vi "Serial Write.vi"(8 "error in (no error)":errorcluster, 9 "Write Buffer":string, 10 "Connection ID":i32, 11 "Gantry in":refnum<class "Gantry.lvclass">) -> (0 "error out":errorcluster, 2 "Bytes written":u32, 3 "Gantry out":refnum<class "Gantry.lvclass">)   [LabVIEW 2023, in "Gantry.lvclass"]
uses:
  Gantry.lvclass
  Gantry.lvclass/Gantry.ctl
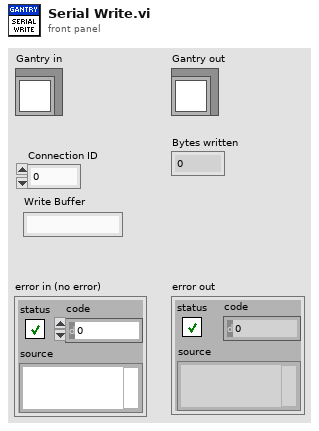
[diagram p1: front panel]
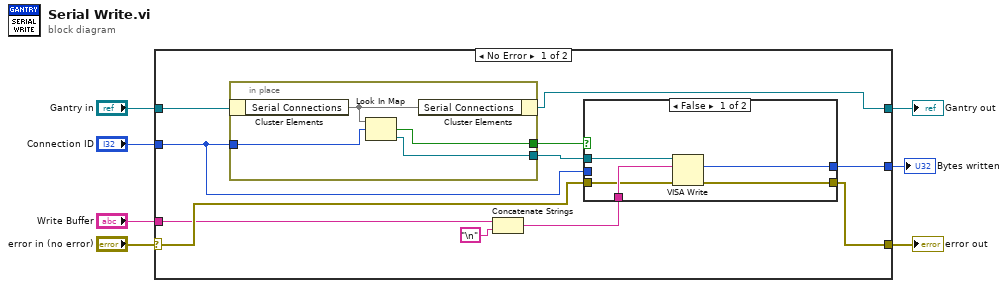
[diagram p0: block diagram]
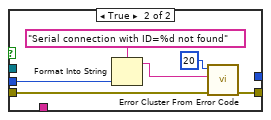
[diagram p2: hidden frame]
diagram:
  n1 = case shown="No Error" "error in (no error)" {
    selector: "error in (no error)" -> [w13 w35]
    tunnel: [w12 w35] -> w6
    tunnel: [w15 w34] -> w4
    tunnel: "Gantry in" -> [w16 w34]
    tunnel: "Connection ID" -> [w14 _]
    tunnel: "Write Buffer" -> [w10 _]
    tunnel: [w11 _] -> w1
    frame No Error {
      n2 = in-place {
        in-place-border: w14 -> [w33]
        in-place-border: [w32] -> w17
        in-place-border: [w31] -> w18
        n3 = in-place-cluster #1(w16) -> ("Serial Connections"=w30:map{i32, refnum<visa-resource-name>})
        n4 = Look In Map(map=w30, key=w33) -> (key not found?=w31:bool, value=w32:refnum<visa-resource-name>)  [unwired: 1 in]
        n5 = in-place-cluster #1("Serial Connections"=w30) -> (w15:refnum<class "Gantry.lvclass">)
      }
      n6 = Concatenate Strings(w10, "\n") -> (w8:string)
      n7 = case shown="False" w18 {
        tunnel: w17 -> [w23 _]
        tunnel: w13 -> [w21 w29]
        tunnel: w14 -> [_ w26]
        tunnel: [w20 w24] -> w12
        tunnel: w8 -> [w22 _]
        tunnel: [w19 _] -> w11
        frame False {
          n8 = VISA Write(VISA resource name=w23, write buffer=w22, error in (no error)=w21) -> (return count=w19:u32, error out=w20:errorcluster)  [unwired: 1 out]
        }
        frame True {
          n9 = Format Into String(format string="Serial connection with ID=%d not found", w26) -> (resulting string=w25:string)  [unwired: 2 in, 1 out]
          n10 = call <vilib>:"Error Cluster From Error Code.vi"("error in (no error)"=w29, "error message (\"\")"=w25, "error code (0)"=20) -> ("error out"=w24:errorcluster)  [unwired: 6 in]
        }
      }
    }
    frame Error {
    }
  }
  "error out" <- w6
  "Gantry out" <- w4
  "Bytes written" <- w1
